vi "Hook Controller.vi"(1 "error in":errorcluster, 2 "Button B":bool, 3 "Button A":bool) -> (0 "error out":errorcluster)   [LabVIEW 2017]
uses:
  <vilib>/Rock Robotics/WPI/Solenoid/WPI_SolenoidValue.ctl
  <vilib>/Rock Robotics/WPI/Solenoid/WPI_SolenoidGetEnum.vi
  <vilib>/Rock Robotics/WPI/Solenoid/WPI_SolenoidSetEnum.vi
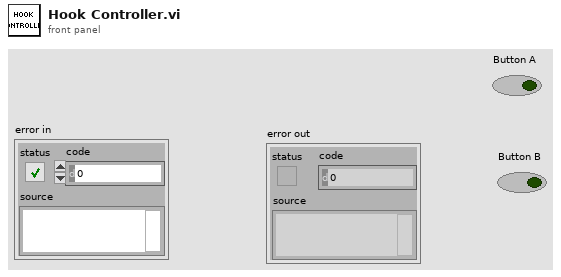
[diagram p1: front panel]
types:
  T1 = typedef "WPI_SolenoidValue.ctl" = enum16{"Off", "On", "Forward", "Reverse"}
  T2 = typedef "WPI_SolenoidDevRef.ctl" = cluster{"DevStatus":errorcluster, "Pneumatics Control Module":u8, "Forward Solenoid Channel":T3, "Reverse Solenoid Channel":T3}
  T3 = typedef "WPI_SolenoidChannel.ctl" = enum8{"Solenoid 0", "Solenoid 1", "Solenoid 2", "Solenoid 3", "Solenoid 4", "Solenoid 5", "Solenoid 6", "Solenoid 7", "Invalid"}
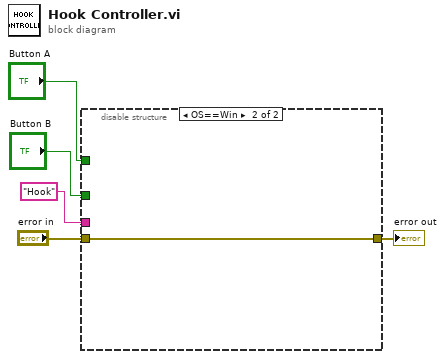
[diagram p0: block diagram]
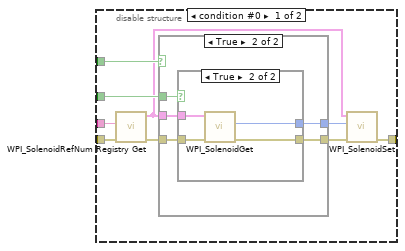
[diagram p2: hidden frame]
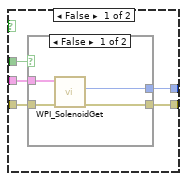
[diagram p3: hidden frame]
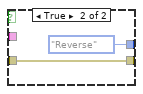
[diagram p4: hidden frame]
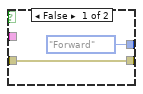
[diagram p5: hidden frame]
diagram:
  n1 = disable-structure shown="OS==Win" {
    disable-tunnel: "Hook" ("refnum name") -> [w14 _]
    disable-tunnel: [w13 w37] -> w4
    disable-tunnel: "Button A" -> [w12 _]
    disable-tunnel: "Button B" -> [w11 _]
    disable-tunnel: "error in" -> [w9 w37]
    frame condition #0 {
      n2 = call <vilib>:"WPI_SolenoidRefNum Registry Get.vi"("error in (no error)"=w9, "refnum name"=w14) -> ("error out"=w8:errorcluster, "SolenoidDevRef"=w10:T2)  [unwired: 8 in]
      n3 = case shown="True" w12 {
        tunnel: w11 -> [w19 w30]
        tunnel: w10 -> [w18 w29]
        tunnel: w8 -> [w17 w27]
        tunnel: [w16 w26] -> w7
        tunnel: [w15 w28] -> w6
        frame False {
          n4 = case shown="False" w19 {
            tunnel: [w22 WPI_SolenoidValue."Reverse" ("Value")] -> w15
            tunnel: w18 -> [w23 _]
            tunnel: w17 -> [w21 w24]
            tunnel: [w20 w24] -> w16
            frame False {
              n5 = call-poly <vilib>:"WPI_SolenoidGet.vi"("error in (no error)"=w21, "SolenoidDevRef"=w23) -> ("error out"=w20:errorcluster, "Value"=w22:T1)  [unwired: 7 in, 1 out]
            }
            frame True {
            }
          }
        }
        frame True {
          n6 = case shown="True" w30 {
            tunnel: w29 -> [_ w36]
            tunnel: [WPI_SolenoidValue."Forward" ("Value") w35] -> w28
            tunnel: w27 -> [w31 w34]
            tunnel: [w31 w33] -> w26
            frame False {
            }
            frame True {
              n7 = call-poly <vilib>:"WPI_SolenoidGet.vi"("error in (no error)"=w34, "SolenoidDevRef"=w36) -> ("error out"=w33:errorcluster, "Value"=w35:T1)  [unwired: 7 in, 1 out]
            }
          }
        }
      }
      n8 = call-poly <vilib>:"WPI_SolenoidSet.vi"("error in (no error)"=w7, "Value"=w6, "SolenoidDevRef"=w10) -> ("error out"=w13:errorcluster)  [unwired: 7 in, 1 out]
    }
    frame condition #1 (active) {
    }
  }
  "error out" <- w4
